vi "MRC IMU Get Euler Angles Portrait.vi"(8 "error in (no error)":errorcluster) -> (0 "error out":errorcluster, 2 "function return":i32, 3 "angles":T1)   [LabVIEW 2026, in "MrcLib.lvlib"]
doc: "MRC_Status MRC_CALLCONV MRC_IMU_GetEulerAnglesPortrait(struct MRC_EulerAngles3d* eulerAngles);"
uses:
  MrcLib.lvlib
  Types/MRC Euler Angles.ctl
  MrcLib.so
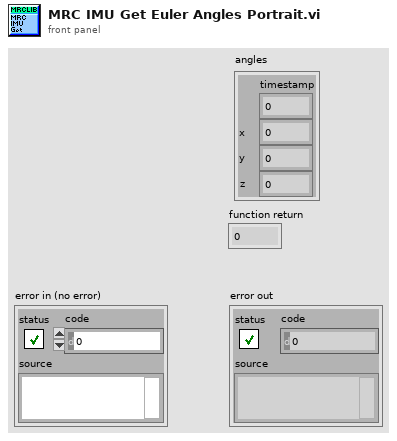
[diagram p1: front panel]
types:
  T1 = typedef "MrcLib.lvlib/MRC Euler Angles.ctl" = cluster{"timestamp":i64, "x":dbl, "y":dbl, "z":dbl}
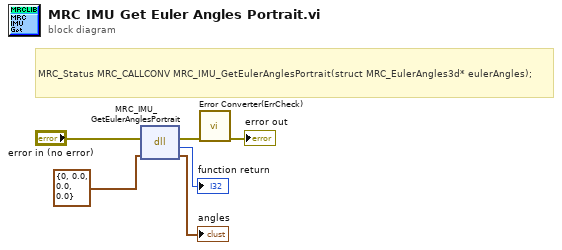
[diagram p0: block diagram]
diagram:
  # "MRC_Status MRC_CALLCONV MRC_IMU_GetEulerAnglesPortrait(struct MRC_EulerAngles3d* eulerAngles);"
  n1 = dll-call lib="MrcLib.*" fn="MRC_IMU_GetEulerAnglesPortrait"(error in="error in (no error)", "eulerAngles"=T1 {"timestamp"=0, "x"=0.0, "y"=0.0, "z"=0.0} ("angles")) -> (error out=w2:errorcluster, →"function return":i32, "eulerAngles"=→"angles":T1)  [unwired: 2 in, 1 out]
  n2 = call "Error Converter(ErrCheck).vi"("error in (no error)"=w2) -> ("error out"=→"error out":errorcluster)  [unwired: 10 in]
